vi "Init_Kamera.vi"(8 "Fehler in":errorcluster, 10 "Kamera":enum16{"Kamera Oben", "Kamera Unten"}(ring), 11 "Kamera in":T1) -> (0 "Fehler out":errorcluster, 3 "Kamera out":T1)   [LabVIEW 2024]
uses:
  Kontaktmontagemodul.exe/1abvi3w/vi.lib/userDefined/High Color/IMAQdx.ctl
  Kontaktmontagemodul.exe/1abvi3w/vi.lib/vision/driver/IMAQdx.llb/IMAQdx Acquisition Mode.ctl
  <resource>/objmgr/imaqdx.rc
  Kontaktmontagemodul.exe/1abvi3w/vi.lib/vision/driver/NI_Vision_Acquisition_Software.lvlib
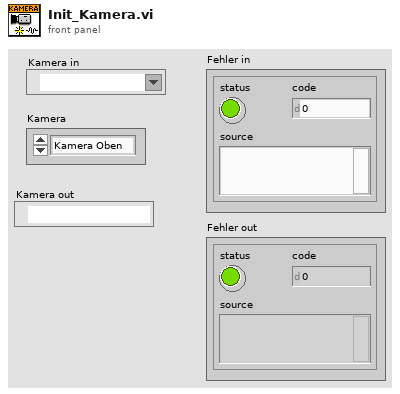
[diagram p1: front panel]
types:
  T1 = typedef "IMAQdx.ctl" = refnum<k21>
  T2 = typedef "NI_Vision_Acquisition_Software.lvlib/IMAQdx Acquisition Mode.ctl" = enum32{"One Shot", "Continuous"}
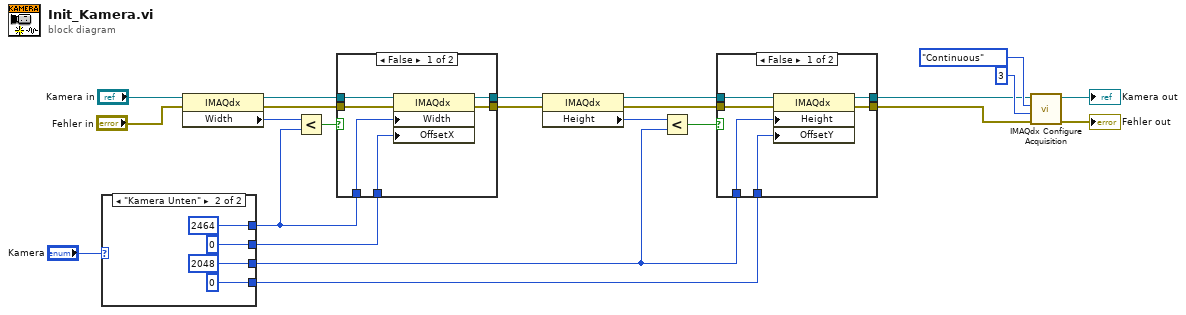
[diagram p0: block diagram]
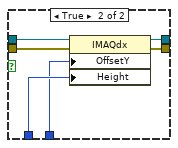
[diagram p2: hidden frame]
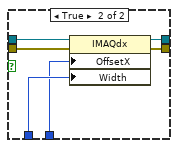
[diagram p3: hidden frame]
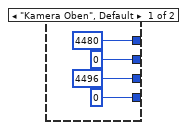
[diagram p4: hidden frame]
diagram:
  n1 = case shown="\"Kamera Unten\"" "Kamera" {
    tunnel: [u32 4480 ("Width") u32 2464 ("Width")] -> w13
    tunnel: [u32 0 ("Width") u32 0 ("Width")] -> w9
    tunnel: [u32 4496 ("Width") u32 2048 ("Width")] -> w3
    tunnel: [u32 0 ("Width") u32 0 ("Width")] -> w2
    frame "Kamera Oben", Default {
    }
    frame "Kamera Unten" {
    }
  }
  n2 = property class="IMAQdx"(reference="Kamera in", error in="Fehler in") -> (reference out=w16:T1, error out=w15:errorcluster, "Width"=w14:u32)
  n3 = Less?(x=w14, y=w13) -> (x < y?=w12:bool)
  n4 = case shown="False" w12 {
    tunnel: w13 -> [w37 w39]
    tunnel: w9 -> [w36 w38]
    tunnel: [w35 w42] -> w11
    tunnel: [w34 w40] -> w10
    tunnel: w16 -> [w33 w43]
    tunnel: w15 -> [w32 w41]
    frame False {
      n5 = property class="IMAQdx"(reference=w33, error in=w32, "Width"=w37, "OffsetX"=w36) -> (reference out=w35:T1, error out=w34:errorcluster)
    }
    frame True {
      n6 = property class="IMAQdx"(reference=w43, error in=w41, "OffsetX"=w38, "Width"=w39) -> (reference out=w42:T1, error out=w40:errorcluster)
    }
  }
  n7 = property class="IMAQdx"(reference=w11, error in=w10) -> (reference out=w6:T1, error out=w8:errorcluster, "Height"=w5:u32)
  n8 = Less?(x=w5, y=w3) -> (x < y?=w4:bool)
  n9 = case shown="False" w4 {
    tunnel: w3 -> [w49 w51]
    tunnel: w2 -> [w48 w50]
    tunnel: [w47 w54] -> w1
    tunnel: [w46 w52] -> w7
    tunnel: w6 -> [w45 w55]
    tunnel: w8 -> [w44 w53]
    frame False {
      n10 = property class="IMAQdx"(reference=w45, error in=w44, "Height"=w49, "OffsetY"=w48) -> (reference out=w47:T1, error out=w46:errorcluster)
    }
    frame True {
      n11 = property class="IMAQdx"(reference=w55, error in=w53, "OffsetY"=w50, "Height"=w51) -> (reference out=w54:T1, error out=w52:errorcluster)
    }
  }
  n12 = call "IMAQdx Configure Acquisition.vi"("error in"=w7, "Number of Buffers"=u32 3, "Continuous?"=IMAQdx_Acquisition_Mode."Continuous", "Session In"=w1) -> ("error out"=→"Fehler out":errorcluster, "Session Out"=→"Kamera out":T1)  [unwired: 6 in]
